vi "Init Rolat.vi"   [LabVIEW 2019]
uses:
  <vilib>/Rock Robotics/WPI/ThirdParty/Phoenix-LabVIEW/Motor Controller/Controls/CTRE_Phoenix_MotorControl_ControlMode.ctl
  <vilib>/Rock Robotics/WPI/ThirdParty/Phoenix-LabVIEW/Motor Controller/Controls/CTRE_Phoenix_MotorControl_NeutralMode.ctl
  <vilib>/Rock Robotics/WPI/ThirdParty/Phoenix-LabVIEW/Motor Controller/Controls/CTRE_Phoenix_MotorControl_FeedbackDevice.ctl
  <vilib>/Rock Robotics/WPI/Solenoid/WPI_SolenoidChannel.ctl
  <vilib>/Rock Robotics/WPI/Solenoid/WPI_SolenoidOpenSingle.vi
types:
  T1 = typedef "WPI_SolenoidChannel.ctl" = enum8{"Solenoid 0", "Solenoid 1", "Solenoid 2", "Solenoid 3", "Solenoid 4", "Solenoid 5", "Solenoid 6", "Solenoid 7", "Invalid"}
  T2 = typedef "CTRE_Phoenix_MotorControl_FeedbackDevice.ctl" = i8
  T3 = typedef "CTRE_Phoenix_MotorControl_NeutralMode.ctl" = enum8{"EEPROMSetting", "Override to Coast", "Override to Brake"}
  T4 = typedef "CTRE_Phoenix_MotorControl_ControlMode.ctl" = u16
  T5 = typedef "WPI_SolenoidDevRef.ctl" = cluster{"DevStatus":errorcluster, "Pneumatics Control Module":u8, "Forward Solenoid Channel":T1, "Reverse Solenoid Channel":T1}
  T6 = typedef "WPI_MotorControlDeviceRef.ctl" = cluster{"DeviceStatus":errorcluster, "Type":T7, "PWM":cluster{"PWM Channel":T8, "DeadBand":T9}, "CAN":cluster{"Device Number":u8, "SetOutput VI Ref":variant, "GetOutput VI Ref":variant, "Enable VI Ref":variant, "Disable VI Ref":variant, "Data":variant}, "Invert":bool, "DIO PWM":cluster{"PWM \"Enable\" Channel":T8, "DIOChannel":T10, "PWM Rate":dbl}}
  T7 = typedef "WPI_MotorControlType.ctl" = enum16{"PWM", "CAN", "DIO PWM"}
  T8 = typedef "FPGA_DIOPWMChannel.ctl" = enum8{"PWM 0", "PWM 1", "PWM 2", "PWM 3", "PWM 4", "PWM 5", "PWM 6", "PWM 7", "PWM 8", "PWM 9", "PWM MXP 0", "PWM MXP 1", "PWM MXP 2", "PWM MXP 3", "PWM MXP 4", "PWM MXP 5", "PWM MXP 6", "PWM MXP 7", "PWM MXP 8", "PWM MXP 9", "Invalid"}
  T9 = typedef "WPI_PWMDeadband.ctl" = cluster{"Name":string, "maxPositivePwm":i32, "minPositivePwm":i32, "centerPwm":i32, "maxNegativePwm":i32, "minNegativePwm":i32, "angularRange":u16}
  T10 = typedef "FPGA_DIOChannel.ctl" = enum8{"DIO 0", "DIO 1", "DIO 2", "DIO 3", "DIO 4", "DIO 5", "DIO 6", "DIO 7", "DIO 8", "DIO 9", "DIO MXP 0", "DIO MXP 1", "DIO MXP 2", "DIO MXP 3", "DIO MXP 4", "DIO MXP 5", "DIO MXP 6", "DIO MXP 7", "DIO MXP 8", "DIO MXP 9", "DIO MXP 10", "DIO MXP 11", "DIO MXP 12", "DIO MXP 13", "DIO MXP 14", "DIO MXP 15", "SPI Port CS1", "SPI Port CS2", "SPI Port CS3", "SPI Port MISO", "SPI Port MOSI", "Invalid"}
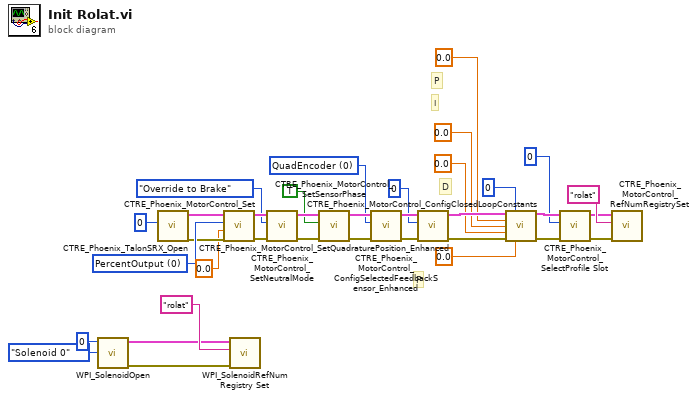
[diagram p0: block diagram]
diagram:
  w25 = T2 0 items=["None"=-1, "QuadEncoder"=0, "Analog"=2, "Tachometer"=4, "Pulse Width Encoded Position"=8, "Sensor Sum (S0 + S1)"=9, "Sensor Difference (D0 - D1)"=10, "Remote Source 0"=11, "Remote Source 1"=12, "Software Emulated"=15] ("Feedback Device")
  w9 = T4 0 items=["PercentOutput"=0, "Position"=1, "Velocity"=2, "Current"=3, "Follower"=5, "MotionProfile"=6, "MotionMagic"=7, "MotionMagicArc"=8, "MotionProfileArc"=10, "Disabled"=15] ("Control Mode")
  # "F"
  # "D"
  # "I"
  # "P"
  n1 = call-poly <vilib>:"WPI_SolenoidOpen.vi"("Solenoid Channel"=WPI_SolenoidChannel."Solenoid 0", "Pneumatics Control Module (0)"=u8 0) -> ("error out"=w3:errorcluster, "SolenoidDevRef"=w4:T5)  [unwired: 8 in]
  n2 = call <vilib>:"CTRE_Phoenix_TalonSRX_Open.vi"("Device Number"=u8 0) -> ("error out"=w7:errorcluster, "CAN Talon SRX Ref"=w11:T6)  [unwired: 9 in]
  n3 = call <vilib>:"CTRE_Phoenix_MotorControl_Set.vi"("error in (no error)"=w7, "Output"=0.0, "Control Mode"=w9, "PhoenixMotorControlDevRef"=w11) -> ("error out"=w29:errorcluster, "PhoenixMotorControlDevRef"=w33:T6)  [unwired: 6 in]
  n4 = call <vilib>:"WPI_SolenoidRefNum Registry Set.vi"("error in (no error)"=w3, "refnum name"="rolat", "SolenoidDevRef"=w4) -> ()  [unwired: 7 in, 2 out]
  n5 = call <vilib>:"CTRE_Phoenix_MotorControl_SetNeutralMode.vi"("error in (no error)"=w29, "Motor Control Neutral Mode"=CTRE_Phoenix_MotorControl_NeutralMode."Override to Brake", "PhoenixMotorControlDevRef"=w33) -> ("error out"=w31:errorcluster, "PhoenixMotorControlDevRef"=w30:T6)  [unwired: 7 in]
  n6 = call <vilib>:"CTRE_Phoenix_MotorControl_SetSensorPhase.vi"("error in (no error)"=w31, "PhaseSensor"=TRUE, "PhoenixMotorControlDevRef"=w30) -> ("error out"=w27:errorcluster, "PhoenixMotorControlDevRef"=w26:T6)  [unwired: 7 in]
  n7 = call <vilib>:"CTRE_Phoenix_MotorControl_ConfigSelectedFeedbackSensor_Enhanced.vi"("error in (no error)"=w27, "Feedback Device"=w25, "PhoenixMotorControlDevRef"=w26) -> ("error out"=w23:errorcluster, "PhoenixMotorControlDevRef"=w24:T6)  [unwired: 7 in]
  n8 = call <vilib>:"CTRE_Phoenix_MotorControl_SetQuadraturePosition_Enhanced.vi"("error in (no error)"=w23, "New Position"=0, "PhoenixMotorControlDevRef"=w24) -> ("error out"=w20:errorcluster, "PhoenixMotorControlDevRef"=w21:T6)  [unwired: 7 in]
  n9 = call <vilib>:"CTRE_Phoenix_MotorControl_ConfigClosedLoopConstants.vi"("PhoenixMotorControlDevRef"=w21, "slotIdx"=0, "P"=0.0, "I"=0.0, "D"=0.0, "error in (no error)"=w20, "F"=0.0) -> ("PhoenixMotorControlDevRef"=w13:T6, "error out"=w14:errorcluster)  [unwired: 7 in]
  n10 = call <vilib>:"CTRE_Phoenix_MotorControl_SelectProfile Slot.vi"("error in (no error)"=w14, "slotIdx"=0, "PhoenixMotorControlDevRef"=w13) -> ("error out"=w8:errorcluster, "PhoenixMotorControlDevRef"=w10:T6)  [unwired: 7 in]
  n11 = call <vilib>:"CTRE_Phoenix_MotorControl_RefNumRegistrySet.vi"("error in (no error)"=w8, "refnum name"="rolat", "PhoenixMotorControlDevRef"=w10) -> ()  [unwired: 7 in, 2 out]
